vi "_Main.vi"   [LabVIEW 2017, in "NavX.lvlib"]
uses:
  NavX.lvlib
  <vilib>/Rock Robotics/WPI/ThirdParty/Sensors/navX/_TypeDefs/FRIC_navX_DeviceNumbersTypeDef.ctl
  <vilib>/Rock Robotics/WPI/ThirdParty/Sensors/navX/_Processing Loop/FRIC_navX_Internal_SPI_ProcessingLoop.vi
  _SHARE ALL/Global Share All/Global_STOP.vi
types:
  T1 = typedef "FRIC_navX_DeviceNumbersTypeDef.ctl" = enum16{"Dev0", "Dev1", "Dev2", "Dev3"}
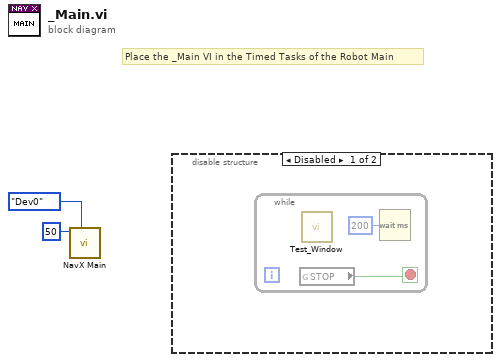
[diagram p0: block diagram]
diagram:
  # "Place the _Main VI in the Timed Tasks of the Robot Main"
  n1 = call-poly <vilib>:"NavX Main.vi"("Device Number"=FRIC_navX_DeviceNumbersTypeDef."Dev0", "Rate (4Hz-200Hz)"=u8 50) -> ()  [unwired: 10 in]
  n2 = disable-structure shown="Disabled" {
    frame Disabled {
      n3 = while {
        stop <- w3 stop-if-true
        n4 = global read "Global_STOP.vi" "STOP"() -> (w3:bool)
        n5 = call <vilib>:"Test_Window.vi"() -> ()  [unwired: 12 in]
        n6 = Wait (ms)(milliseconds to wait=u32 200) -> ()  [unwired: 1 out]
      }
    }
    frame Enabled {
    }
  }
